vi "Read value.vi"(8 "error in (no error)":errorcluster, 11 "AD9850 in":refnum<class "AD9850.lvclass">) -> (0 "error out":errorcluster, 2 "value":string, 3 "AD9850 out":refnum<class "AD9850.lvclass">)   [LabVIEW 2014, in "LabVIEW Universal Transcriptor AD9850.lvlib" / "AD9850.lvclass"]
uses:
  AD9850.lvclass
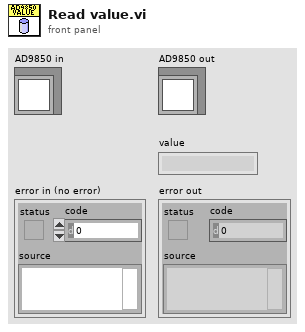
[diagram p1: front panel]
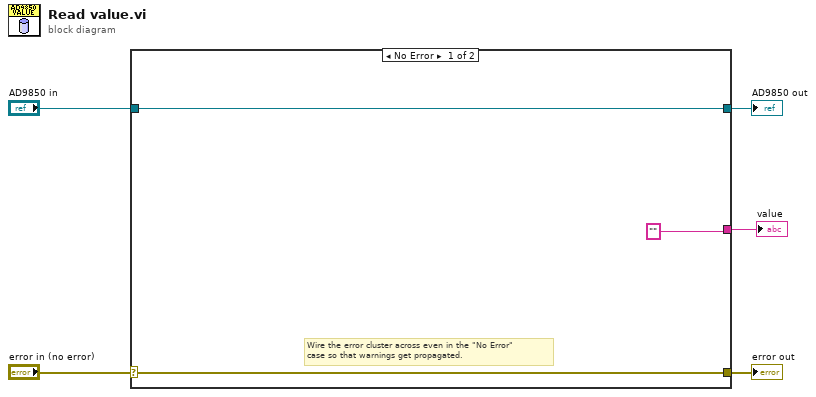
[diagram p0: block diagram]
diagram:
  n1 = case shown="No Error" "error in (no error)" {
    selector: "error in (no error)" -> [w7 w10]
    tunnel: [w7 w10] -> w4
    tunnel: [w8 w9] -> w2
    tunnel: "AD9850 in" -> [w8 w9]
    tunnel: ["" _] -> w1
    frame No Error {
      # "Wire the error cluster across even in the \"No Error\"\ncase so that warnings get propagated."
    }
    frame Error {
    }
  }
  "error out" <- w4
  "AD9850 out" <- w2
  "value" <- w1
